vi "_Destroy.vi"(8 "error in (no error)":errorcluster, 11 "Spectrometer iHR320 in":refnum<class "Spectrometer ActiveX.lvclass">) -> (0 "error out":errorcluster)   [LabVIEW 2015, in "Spectrometer ActiveX.lvclass"]
doc: "Superclass destructor: close all handles to and release all resources associated with this Instrument, then deallocate it. \n\nIMPORTANT: when destroying a class that inherits from Instrument, destroy your subclass first, and call the parent Instrument::_Destroy.vi LAST. This ensures your subclass destructor operates on a valid Instrument while it releases its resources."
uses:
  Spectrometer ActiveX.lvclass
  Spectrometer ActiveX.lvclass/Spectrometer ActiveX.ctl
  Utility Classes/Scannable/Scannable.lvclass
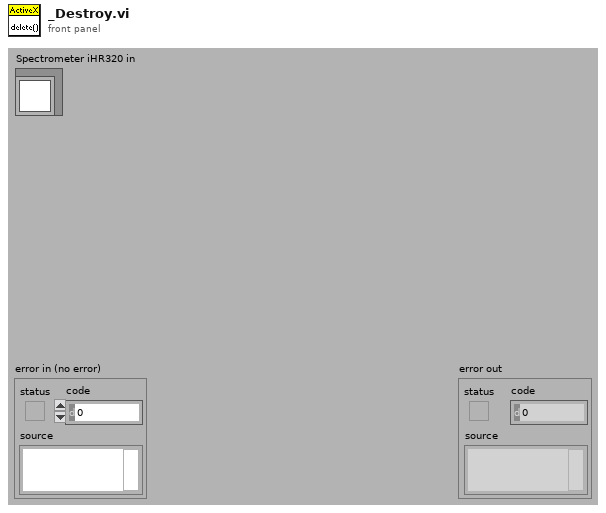
[diagram p1: front panel]
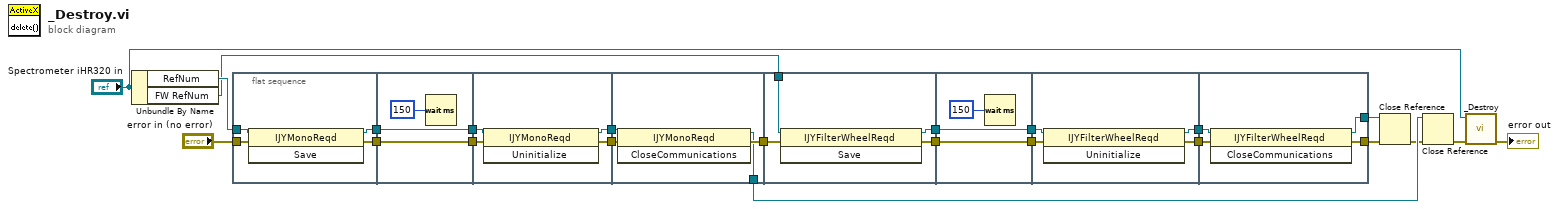
[diagram p0: block diagram]
diagram:
  n1 = Unbundle By Name("Spectrometer iHR320 in") -> ("RefNum"=w20:refnum<k7>, "FW RefNum"=w10:refnum<k7>)
  n2 = flat-sequence {
    tunnel: w20 -> [w27]
    tunnel: "error in (no error)" -> [w26]
    tunnel: [w25] -> w18
    tunnel: [w24] -> w17
    tunnel: w18 -> [w30]
    tunnel: w17 -> [w29]
    tunnel: [w30] -> w13
    tunnel: [w29] -> w12
    tunnel: [w34] -> w15
    tunnel: [w33] -> w14
    tunnel: w13 -> [w32]
    tunnel: w12 -> [w31]
    tunnel: [w37] -> w16
    tunnel: w15 -> [w36]
    tunnel: w14 -> [w35]
    tunnel: [w38] -> w11
    tunnel: w11 -> [w41]
    tunnel: w10 -> [w42]
    tunnel: [w40] -> w8
    tunnel: [w39] -> w6
    tunnel: [w44] -> w9
    tunnel: w8 -> [w44]
    tunnel: [w43] -> w7
    tunnel: w6 -> [w43]
    tunnel: w9 -> [w49]
    tunnel: w7 -> [w48]
    tunnel: [w47] -> w5
    tunnel: [w46] -> w4
    tunnel: w5 -> [w53]
    tunnel: w4 -> [w52]
    tunnel: [w51] -> w3
    tunnel: [w50] -> w2
    frame #0 {
      n3 = invoke class="IJYMonoReqd" method="Save"(reference=w27, error in=w26) -> (reference out=w24:refnum<k7>, error out=w25:errorcluster)  [unwired: 1 in, 1 out]
    }
    frame #1 {
      n4 = Wait (ms)(milliseconds to wait=u32 150) -> ()  [unwired: 1 out]
    }
    frame #2 {
      n5 = invoke class="IJYMonoReqd" method="Uninitialize"(reference=w31, error in=w32) -> (reference out=w33:refnum<k7>, error out=w34:errorcluster)  [unwired: 1 in, 1 out]
    }
    frame #3 {
      n6 = invoke class="IJYMonoReqd" method="CloseCommunications"(reference=w35, error in=w36) -> (reference out=w37:refnum<k7>, error out=w38:errorcluster)  [unwired: 1 in, 1 out]
    }
    frame #4 {
      n7 = invoke class="IJYFilterWheelReqd" method="Save"(reference=w42, error in=w41) -> (reference out=w40:refnum<k7>, error out=w39:errorcluster)  [unwired: 1 in, 1 out]
    }
    frame #5 {
      n8 = Wait (ms)(milliseconds to wait=u32 150) -> ()  [unwired: 1 out]
    }
    frame #6 {
      n9 = invoke class="IJYFilterWheelReqd" method="Uninitialize"(reference=w49, error in=w48) -> (reference out=w47:refnum<k7>, error out=w46:errorcluster)  [unwired: 1 in, 1 out]
    }
    frame #7 {
      n10 = invoke class="IJYFilterWheelReqd" method="CloseCommunications"(reference=w53, error in=w52) -> (reference out=w51:refnum<k7>, error out=w50:errorcluster)  [unwired: 1 in, 1 out]
    }
  }
  n11 = Close Reference(reference=w3, error in (no error)=w2) -> (error out=w1:errorcluster)
  n12 = Close Reference(reference=w16, error in (no error)=w1) -> (error out=w22:errorcluster)
  n13 = call-parent "_Destroy.vi"("error in (no error)"=w22, "Instrument in"="Spectrometer iHR320 in") -> ("error out"=→"error out":errorcluster)  [unwired: 9 in]
